vi "Fetch_chirp_waveform .vi"(8 "error in (no error)":errorcluster, 9 "Maximum Time (10000ms)":u32=10000, 10 "Channel (0:Channel1)":u16(ring) items=["Channel1", "Channel2", "Channel3", "Channel4", "Math1", "Math2", "Math3", "Math3", "Reference1", "Reference2", "Reference3", "Reference4"], 11 "VISA resource name":refnum<visa-resource-name>) -> (0 "error out":errorcluster, 1 "meas time":u32, 2 "Waveform Data":waveform(dbl)(graph)={"t0"=timestamp(3.694502999999883e-07 s since 1904-01-01), "dt"=5e-07, "Y"=array[10000 elements]}, 3 "VISA resource name out":refnum<visa-resource-name>)   [LabVIEW 2011]
doc: "Returns the waveform that an oscilloscope acquires for a channel you specify. An acquisition that you initiate before calling this VI generates the waveform.\n\nYou first enable channels with the Configure Channel VI. Then you use the Initiate VI to start an acquisition on the enabled channels. An oscilloscope concurrently acquires waveforms for these channels. You must call the Fetch Waveform VI separately to obtain waveforms for each enabled channel. However, you also can call the Read Waveform VI instead of using the above low-level VIs.\n\n<B>Note:</B> Use the Fetch Waveform VI only with other low-level VIs, such as the Initiate VI, the Abort VI, and the Fetch Waveform Measurement VI. High-level VIs such as the Read Waveform VI automatically incorporate the functions of the Initiate VI and the Fetch Waveform VI. The Fetch Waveform VI does not check the status of an instrument."
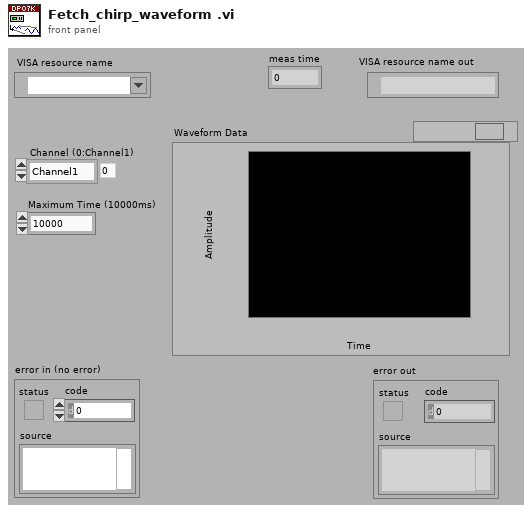
[diagram p1: front panel]
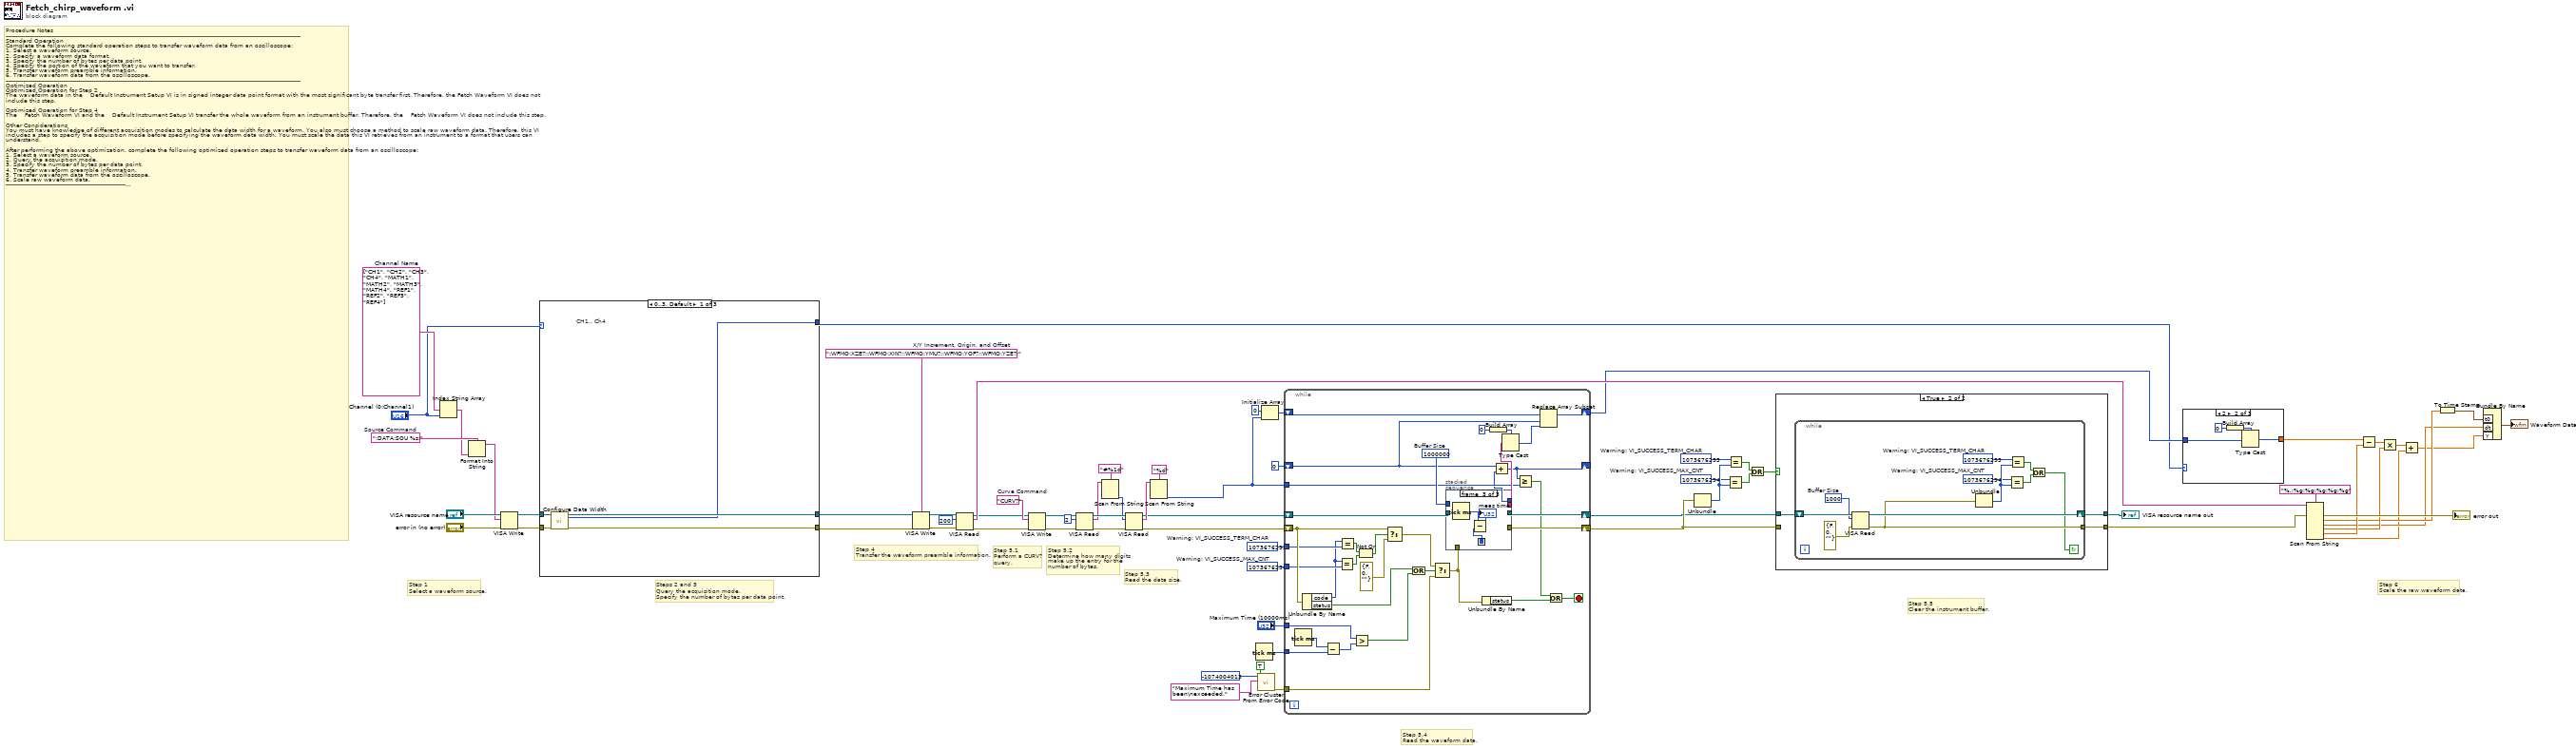
[diagram p0: block diagram]
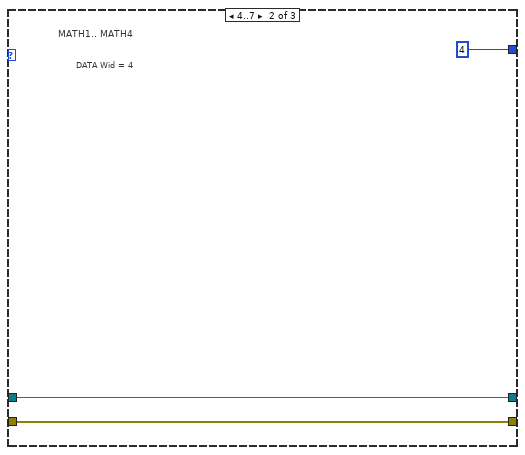
[diagram p2: hidden frame]
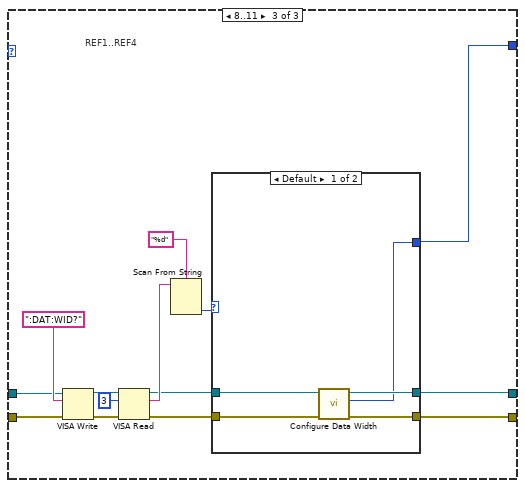
[diagram p3: hidden frame]
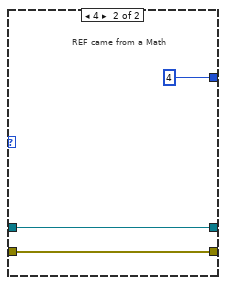
[diagram p4: hidden frame]
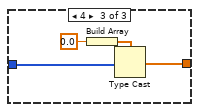
[diagram p6: hidden frame]
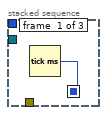
[diagram p8: hidden frame]
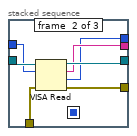
[diagram p9: hidden frame]
diagram:
  w32 = string[] ["CH1", "CH2", "CH3", "CH4", "MATH1", "MATH2", "MATH3", "MATH4", "REF1", "REF2", "REF3", "REF4"]  # Channel Name
  w38 = 1073676294  # Warning: VI_SUCCESS_MAX_CNT
  w39 = 1073676293  # Warning: VI_SUCCESS_TERM_CHAR
  w42 = 1073676294  # Warning: VI_SUCCESS_MAX_CNT
  w41 = 1073676293  # Warning: VI_SUCCESS_TERM_CHAR
  w63 = "CURV?"  # Curve Command
  w68 = ":DATA:SOU %s;"  # Source Command
  w27 = ":WFMO:XZE?;:WFMO:XIN?;:WFMO:YMU?;:WFMO:YOF?;:WFMO:YZE?;"  # X/Y Increment, Origin, and Offset
  # "Step 1       \nSelect a waveform source."
  # "Steps 2 and 3\nQuery the acquisition mode. \nSpecify the number of bytes per data point."
  # "Step 6    \nScale the raw waveform data."
  # "Step 5.5    \nClear the instrument buffer."
  # "Step 5.4   \nRead the waveform data."
  # "Step 5.3      \nRead the data size."
  # "Step 5.2      \nDetermine how many digits\nmake up the entry for the \nnumber of bytes."
  # "Step 5.1      \nPerform a CURV?\nquery."
  # "Step 4\nTransfer the waveform preamble information."
  # "Procedure Notes\n-----------------------------------------------------------------------------------------------------------------------------------------------------------\nStandard Operation\nComplete the following standard operation steps to transfer waveform data from an oscilloscope:\n1. Select a waveform source.\n2. Specify a waveform data format.\n3. Specify the number of bytes per data point.\n4. Specify the portion of the waveform that you want to transfer.\n5. Transfer waveform preamble information.\n6. Transfer waveform data from the oscilloscope.\n-----------------------------------------------------------------------------------------------------------------------------------------------------------\nOptimized Operation\nOptimized Operation for Step 2\nThe waveform data in the    Default Instrument Setup VI is in signed integer data point format with the most significant byte transfer first. Therefore, the Fetch Waveform VI does not include this step.\n\nOptimized Operation for Step 4 \nThe    Fetch Waveform VI and the    Default Instrument Setup VI transfer the whole waveform from an instrument buffer. Therefore, the    Fetch Waveform VI does not include this step.\n\nOther Considerations\nYou must have knowledge of different acquisition modes to calculate the data width for a waveform. You also must choose a method to scale raw waveform data. Therefore, this VI includes a step to specify the acquisition mode before specifying the waveform data width. You must scale the data this VI retrieves from an instrument to a format that users can understand.\n\nAfter performing the above optimization, complete the following optimized operation steps to transfer waveform data from an oscilloscope:\n1. Select a waveform source.\n2. Query the acquisition mode.\n3. Specify the number of bytes per data point.\n4. Transfer waveform preamble information.\n5. Transfer waveform data from the oscilloscope.\n6. Scale raw waveform data.\n-----------------------------------------------------------------------------------------------------------------------------------------------------------\nDetailed Steps\nThe following steps detail the behavior of this VI:\n1. Select a waveform source. \n2. Query and determine the acquisition mode. A correct determination is critical to steps 3 and 6.\n    -----------------------------------------------\n    Acquisition Mode |  Data Width   \n    -----------------------------------------------\n    Normal                       |   1                      \n    -----------------------------------------------\n    Peak Detect               |   1                      \n    -----------------------------------------------\n    Hi Res                        |   2                      \n    -----------------------------------------------\n    Envelope                   |   1                      \n    ----------------------------------------------- \n    Average                    |   2                      \n    -----------------------------------------------\n3. Specify the number of bytes per data point. For the Hi Res or Average acquisition modes, set the data width to 2. For all other acquisition modes, set the data width to 1.\n4. Transfer the waveform preamble information. Necessary preamble information includes XZero, XIncrement, YMultiplier, YOffset, and YZero. This VI uses XZero and XIncrement to configure the x-axis of output waveforms and uses YMultiplier, YOffset, and YZero to scale data values. This VI then parses the return string of the preamble query in step 6.\n5. Transfer waveform data from the oscilloscope.\n    5.1 Perform a CURV? query.\n    5.2 Determine how many digits make up the entry for the number of bytes.\n    5.3 Read the data size.\n    5.4 Call the VISA Read VI repeatedly with a buffer size of 10000 until you obtain as much data as the data size specifies. Use      an 8-bit array to store the raw waveform data you obtain. \n    5.5 Continue reading the data remaining in the instrument buffer until the buffer is empty.\n6. Scale the raw waveform data.\n    6.1 Cast the waveform data to a 16-bit array if the data width is 2. Split the waveform data into a minimum and a maximum data array if the acquisition mode is Peak Detect or Envelope. This VI skips this step if the data width is 1.\n    6.2 Parse the preamble information.\n    6.3 Scale the waveform data according to the following formula:\n          Data_Value_in_units = (Raw_Data_Value - YOffset) * YMultiplier + YZero\n          The resulting waveform data has a unit of volts.\n    6.4 Build a waveform graph."
  n1 = Index String Array(1:"Channel (0:Channel1)", 2:w32) -> (0:w67:string)  [unwired: 1 in]
  n2 = Format Into String(format string=w68, w67) -> (resulting string=w29:string)  [unwired: 2 in, 1 out]
  n3 = VISA Write(VISA resource name="VISA resource name", write buffer=w29, error in (no error)="error in (no error)") -> (VISA resource name out=w21:refnum<visa-resource-name>, error out=w20:errorcluster)  [unwired: 1 out]
  n4 = case shown="0..3, Default" "Channel (0:Channel1)" {
    tunnel: w21 -> [w73 w76 w85]
    tunnel: w20 -> [w72 w75 w86]
    tunnel: [w71 w76 w79] -> w2
    tunnel: [w70 w75 w78] -> w1
    tunnel: [w69 u32 4 ("byte count") w77] -> w5
    frame 0..3, Default {
      # "CH1.. Ch4"
      n5 = call "Configure Data Width.vi"("error in (no error)"=w72, "VISA resource name"=w73) -> ("error out"=w70:errorcluster, "Width"=w69:i32, "VISA resource name out"=w71:refnum<visa-resource-name>)  [unwired: 7 in]
    }
    frame 4..7 {
      # "DATA Wid = 4"
      # "MATH1.. MATH4"
    }
    frame 8..11 {
      # "REF1..REF4"
      n6 = VISA Write(VISA resource name=w85, write buffer=":DAT:WID?", error in (no error)=w86) -> (VISA resource name out=w90:refnum<visa-resource-name>, error out=w89:errorcluster)  [unwired: 1 out]
      n7 = VISA Read(VISA resource name=w90, byte count=u32 3, error in (no error)=w89) -> (VISA resource name out=w81:refnum<visa-resource-name>, read buffer=w84:string, error out=w80:errorcluster)  [unwired: 1 out]
      n8 = Scan From String(format string="%d", input string=w84) -> (output 1=w82:i32)  [unwired: 3 in, 3 out]
      n9 = case shown="Default" w82 {
        tunnel: w81 -> [w95 w98]
        tunnel: w80 -> [w94 w97]
        tunnel: [w93 w98] -> w79
        tunnel: [w92 w97] -> w78
        tunnel: [w91 u32 4 ("byte count")] -> w77
        frame Default {
          n10 = call "Configure Data Width.vi"("error in (no error)"=w94, "VISA resource name"=w95) -> ("error out"=w92:errorcluster, "Width"=w91:i32, "VISA resource name out"=w93:refnum<visa-resource-name>)  [unwired: 7 in]
        }
        frame 4 {
          # "REF came from a Math"
        }
      }
    }
  }
  n11 = VISA Write(VISA resource name=w2, write buffer=w27, error in (no error)=w1) -> (VISA resource name out=w65:refnum<visa-resource-name>, error out=w64:errorcluster)  [unwired: 1 out]
  n12 = VISA Read(VISA resource name=w65, byte count=u32 200, error in (no error)=w64) -> (VISA resource name out=w18:refnum<visa-resource-name>, read buffer=w53:string, error out=w17:errorcluster)  [unwired: 1 out]
  n13 = VISA Write(VISA resource name=w18, write buffer=w63, error in (no error)=w17) -> (VISA resource name out=w19:refnum<visa-resource-name>, error out=w62:errorcluster)  [unwired: 1 out]
  n14 = VISA Read(VISA resource name=w19, byte count=u32 2, error in (no error)=w62) -> (VISA resource name out=w59:refnum<visa-resource-name>, read buffer=w57:string, error out=w58:errorcluster)  [unwired: 1 out]
  n15 = Scan From String(format string="#%1d", input string=w57) -> (output 1=w56:i32)  [unwired: 3 in, 3 out]
  n16 = VISA Read(VISA resource name=w59, byte count=w56, error in (no error)=w58) -> (VISA resource name out=w16:refnum<visa-resource-name>, read buffer=w54:string, error out=w15:errorcluster)  [unwired: 1 out]
  n17 = Scan From String(format string="%d", input string=w54) -> (output 1=w49:i32)  [unwired: 3 in, 3 out]
  n18 = Tick Count (ms)() -> (millisecond timer value=w8:u32)
  n19 = call <vilib>:"Error Cluster From Error Code.vi"("show call chain? (False)"=TRUE, "error message (\"\")"="Maximum Time has been\nexceeded." ("error message (\"\")"), "error code (0)"=-1074004013) -> ("error out"=w6:errorcluster)  [unwired: 6 in]
  n20 = Initialize Array(i8 0 ("element"), w49) -> (w47:i8[])
  n21 = while {
    shift-right: [w131] -> w3
    shift-left: w16 -> [w133]
    shift-right: [w130] -> w4
    shift-left: w15 -> [w120]
    shift-right: [w126] -> w37
    shift-left: w47 -> [w127]
    tunnel: w49 -> [w124]
    shift-right: [w121] -> _
    shift-left: 0 -> [w122]
    tunnel: w39 -> [w119]
    tunnel: w38 -> [w118]
    tunnel: w8 -> [w112]
    tunnel: "Maximum Time (10000ms)" -> [w111]
    tunnel: w6 -> [w106]
    stop <- w102 stop-if-true
    w132 = 1000000  # Buffer Size
    n22 = Tick Count (ms)() -> (millisecond timer value=w113:u32)
    n23 = Unbundle By Name(w120) -> ("code"=w117:i32, "status"=w105:bool)
    n24 = Subtract(x=w113, y=w112) -> (x-y=w110:u32)
    n25 = Equal?(x=w117, y=w118) -> (x = y?=w115:bool)
    n26 = Equal?(x=w117, y=w119) -> (x = y?=w116:bool)
    n27 = Greater?(x=w111, y=w110) -> (0:w104:bool)
    n28 = Not Or(1:w115, 2:w116) -> (0:w114:bool)
    n29 = Select(t=w120, s=w114, f=errorcluster {"status"=FALSE, "code"=0, "source"=""} ("error in (no error)")) -> (s? t:f=w107:errorcluster)
    n30 = Or(x=w105, y=w104) -> (x .or. y?=w108:bool)
    n31 = Select(t=w107, s=w108, f=w106) -> (s? t:f=w101:errorcluster)
    n32 = stacked-sequence {
      seq-local: [w134 _ _] -> [_ _ w143]
      tunnel: w133 -> [_ w141 _]
      tunnel: w132 -> [_ w140 _]
      tunnel: [_ w139 _] -> w131
      tunnel: [_ w138 _] -> w130
      tunnel: [_ w137 _] -> w125
      tunnel: [_ w136 _] -> w99
      tunnel: w101 -> [_ w135 _]
      frame #0 {
        n33 = Tick Count (ms)() -> (millisecond timer value=w134:u32)
      }
      frame #1 {
        n34 = VISA Read(VISA resource name=w141, byte count=w140, error in (no error)=w135) -> (VISA resource name out=w139:refnum<visa-resource-name>, read buffer=w137:string, return count=w136:u32, error out=w138:errorcluster)
      }
      frame #2 {
        n35 = Tick Count (ms)() -> (millisecond timer value=w144:u32)
        n36 = Subtract(x=w144, y=w143) -> (x-y=→"meas time":u32)
      }
    }
    n37 = Unbundle By Name(w101) -> ("status"=w100:bool)
    n38 = Build Array(i8 0) -> (w129:i8[])
    n39 = Add(x=w122, y=w99) -> (x+y=w121:u32)
    n40 = Type Cast(type=w129, x=w125) -> (*(type *) &x=w123:i8[])
    n41 = Greater Or Equal?(x=w121, y=w124) -> (x >= y?=w103:bool)
    n42 = Replace Array Subset(array=w127, new element=w123, index=w122) -> (w126:i8[])
    n43 = Or(x=w103, y=w100) -> (x .or. y?=w102:bool)
  }
  n44 = Unbundle(w4) -> ("code"=w43:i32)  [unwired: 2 out]
  n45 = Equal?(x=w42, y=w43) -> (x = y?=w45:bool)
  n46 = Equal?(x=w41, y=w43) -> (x = y?=w46:bool)
  n47 = Or(x=w46, y=w45) -> (x .or. y?=w44:bool)
  n48 = case shown="True" w44 {
    tunnel: w3 -> [w146 w149]
    tunnel: w4 -> [w145 _]
    tunnel: [w146 w148] -> w50
    tunnel: [w145 w147] -> w52
    frame False {
    }
    frame True {
      n49 = while {
        shift-right: [w159] -> w148
        shift-left: w149 -> [w160]
        tunnel: [w152] -> w147
        stop <- w151 continue-if-true
        w154 = 1073676294  # Warning: VI_SUCCESS_MAX_CNT
        w153 = 1073676293  # Warning: VI_SUCCESS_TERM_CHAR
        w158 = u32 1000  # Buffer Size
        n50 = VISA Read(VISA resource name=w160, byte count=w158, error in (no error)=errorcluster {"status"=FALSE, "code"=0, "source"=""}) -> (VISA resource name out=w159:refnum<visa-resource-name>, error out=w152:errorcluster)  [unwired: 2 out]
        n51 = Unbundle(w152) -> ("code"=w155:i32)  [unwired: 2 out]
        n52 = Equal?(x=w154, y=w155) -> (x = y?=w156:bool)
        n53 = Equal?(x=w153, y=w155) -> (x = y?=w157:bool)
        n54 = Or(x=w157, y=w156) -> (x .or. y?=w151:bool)
      }
    }
  }
  "VISA resource name out" <- w50
  n55 = case shown="2" w5 {
    tunnel: w37 -> [w161 w163 w167]
    tunnel: [w161 w162 w166] -> w25
    frame 1, Default {
    }
    frame 2 {
      n56 = Build Array(i16 0 ("element")) -> (w164:i16[])
      n57 = Type Cast(type=w164, x=w163) -> (*(type *) &x=w162:i16[])
    }
    frame 4 {
      n58 = Build Array(sgl 0.0 ("element")) -> (w168:sgl[])
      n59 = Type Cast(type=w168, x=w167) -> (*(type *) &x=w166:sgl[])
    }
  }
  n60 = Scan From String(format string="%.;%g;%g;%g;%g;%g", input string=w53, error in=w52) -> (error out=→"error out":errorcluster, output 1=w24:dbl, output 2=w22:dbl, output 3=w33:dbl, output 4=w34:dbl, output 5=w13:dbl)  [unwired: 6 in, 2 out]
  n61 = Subtract(x=w25, y=w34) -> (x-y=w35:dbl[])
  n62 = Multiply(x=w35, y=w33) -> (x*y=w14:dbl[])
  n63 = Add(x=w14, y=w13) -> (x+y=w12:dbl[])
  n64 = To Time Stamp(1:w24) -> (0:w23:timestamp)
  n65 = Bundle By Name ("Build Waveform")("t0"=w23, "dt"=w22, "Y"=w12) -> (→"Waveform Data":waveform(dbl))  [unwired: 1 in]
